vi "2013_01_05 Durability8 Main debug.vi"() -> ()   [LabVIEW 2011]
uses:
  MotorTypeDef.ctl
  <vilib>/DAQmx/write.llb/DAQmx Write (Counter Time 1Chan 1Samp).vi
  <vilib>/DAQmx/read.llb/DAQmx Read (Analog 1D Wfm NChan NSamp).vi
  <vilib>/Utility/TradDaqScaling.llb/Convert Thermistor Reading (waveform).vi
  <vilib>/DAQmx/miscellaneous.llb/DAQmx Fill In Error Info.vi
  <vilib>/measure/madcrms.llb/Averaged DC-RMS for N Chan.vi
  <vilib>/measure/NI_MAPro.lvlib
  Program Files/National Instruments/LabVIEW 2011/resource/objmgr/daqmx.rc
panel:
  out "size(s)":i32
  out "error out":errorcluster
  out "main":i32
  out "Voltages":waveform(dbl)[](graph)
  out "Currents":waveform(dbl)[](graph)
  in  "Motor 8":T1 {"Elapsed Time" format="%<%H:%M:%S>t"; "Efficiency" format="%#_3g%%"; "Supply Voltage (V)" format="%#_3f"; "Power Output (W)" format="%#_3g"; "Power Usage (W)" format="%#_3g"; "Torque (mNm)" format="%#_3g"; "RPM" scale=0.0..40000.0 scale format="%#.6p"}
  in  "Motor 7":T1 {"Elapsed Time" format="%<%H:%M:%S>t"; "Efficiency" format="%#_3g%%"; "Supply Voltage (V)" format="%#_3f"; "Power Output (W)" format="%#_3g"; "Power Usage (W)" format="%#_3g"; "Torque (mNm)" format="%#_3g"; "RPM" scale=0.0..40000.0 scale format="%#.6p"}
  in  "Motor 6":T1 {"Elapsed Time" format="%<%H:%M:%S>t"; "Efficiency" format="%#_3g%%"; "Supply Voltage (V)" format="%#_3f"; "Power Output (W)" format="%#_3g"; "Power Usage (W)" format="%#_3g"; "Torque (mNm)" format="%#_3g"; "RPM" scale=0.0..40000.0 scale format="%#.6p"}
  in  "Motor 5":T1 {"Elapsed Time" format="%<%H:%M:%S>t"; "Efficiency" format="%#_3g%%"; "Supply Voltage (V)" format="%#_3f"; "Power Output (W)" format="%#_3g"; "Power Usage (W)" format="%#_3g"; "Torque (mNm)" format="%#_3g"; "RPM" scale=0.0..40000.0 scale format="%#.6p"}
  in  "Motor 4":T1 {"Elapsed Time" format="%<%H:%M:%S>t"; "Efficiency" format="%#_3g%%"; "Supply Voltage (V)" format="%#_3f"; "Power Output (W)" format="%#_3g"; "Power Usage (W)" format="%#_3g"; "Torque (mNm)" format="%#_3g"; "RPM" scale=0.0..40000.0 scale format="%#.6p"}
  in  "Motor 3":T1 {"Elapsed Time" format="%<%H:%M:%S>t"; "Efficiency" format="%#_3g%%"; "Supply Voltage (V)" format="%#_3f"; "Power Output (W)" format="%#_3g"; "Power Usage (W)" format="%#_3g"; "Torque (mNm)" format="%#_3g"; "RPM" scale=0.0..40000.0 scale format="%#.6p"}
  in  "Motor 2":T1 {"Elapsed Time" format="%<%H:%M:%S>t"; "Efficiency" format="%#_3g%%"; "Supply Voltage (V)" format="%#_3f"; "Power Output (W)" format="%#_3g"; "Power Usage (W)" format="%#_3g"; "Torque (mNm)" format="%#_3g"; "RPM" scale=0.0..40000.0 scale format="%#.6p"}
  in  "Motor 1":T1 {"Elapsed Time" format="%<%H:%M:%S>t"; "Efficiency" format="%#_3g%%"; "Supply Voltage (V)" format="%#_3f"; "Power Output (W)" format="%#_3g"; "Power Usage (W)" format="%#_3g"; "Torque (mNm)" format="%#_3g"; "RPM" scale=0.0..40000.0 scale format="%#.6p"}
  out "Motor Temp":dbl(slide) scale=90.0..110.0
  out "Tank Temp":dbl(slide) scale=90.0..110.0
  out "RMS Voltages":waveform(dbl)[](graph)
  out "RMS Currents":waveform(dbl)[](graph)
  in  "Temp Probe\nOn Motor":dbl=1.0
  out "loop time (ms)":u32
  in  "stop":bool
  in  "Unlock PWM":bool=TRUE
  in  "PWM 2":dbl(slide)=100.0 min=0.0 max=100.0 step=5.0 scale=0.0..100.0
  in  "PWM 1":dbl(slide) min=0.0 max=100.0 step=5.0 scale=0.0..100.0
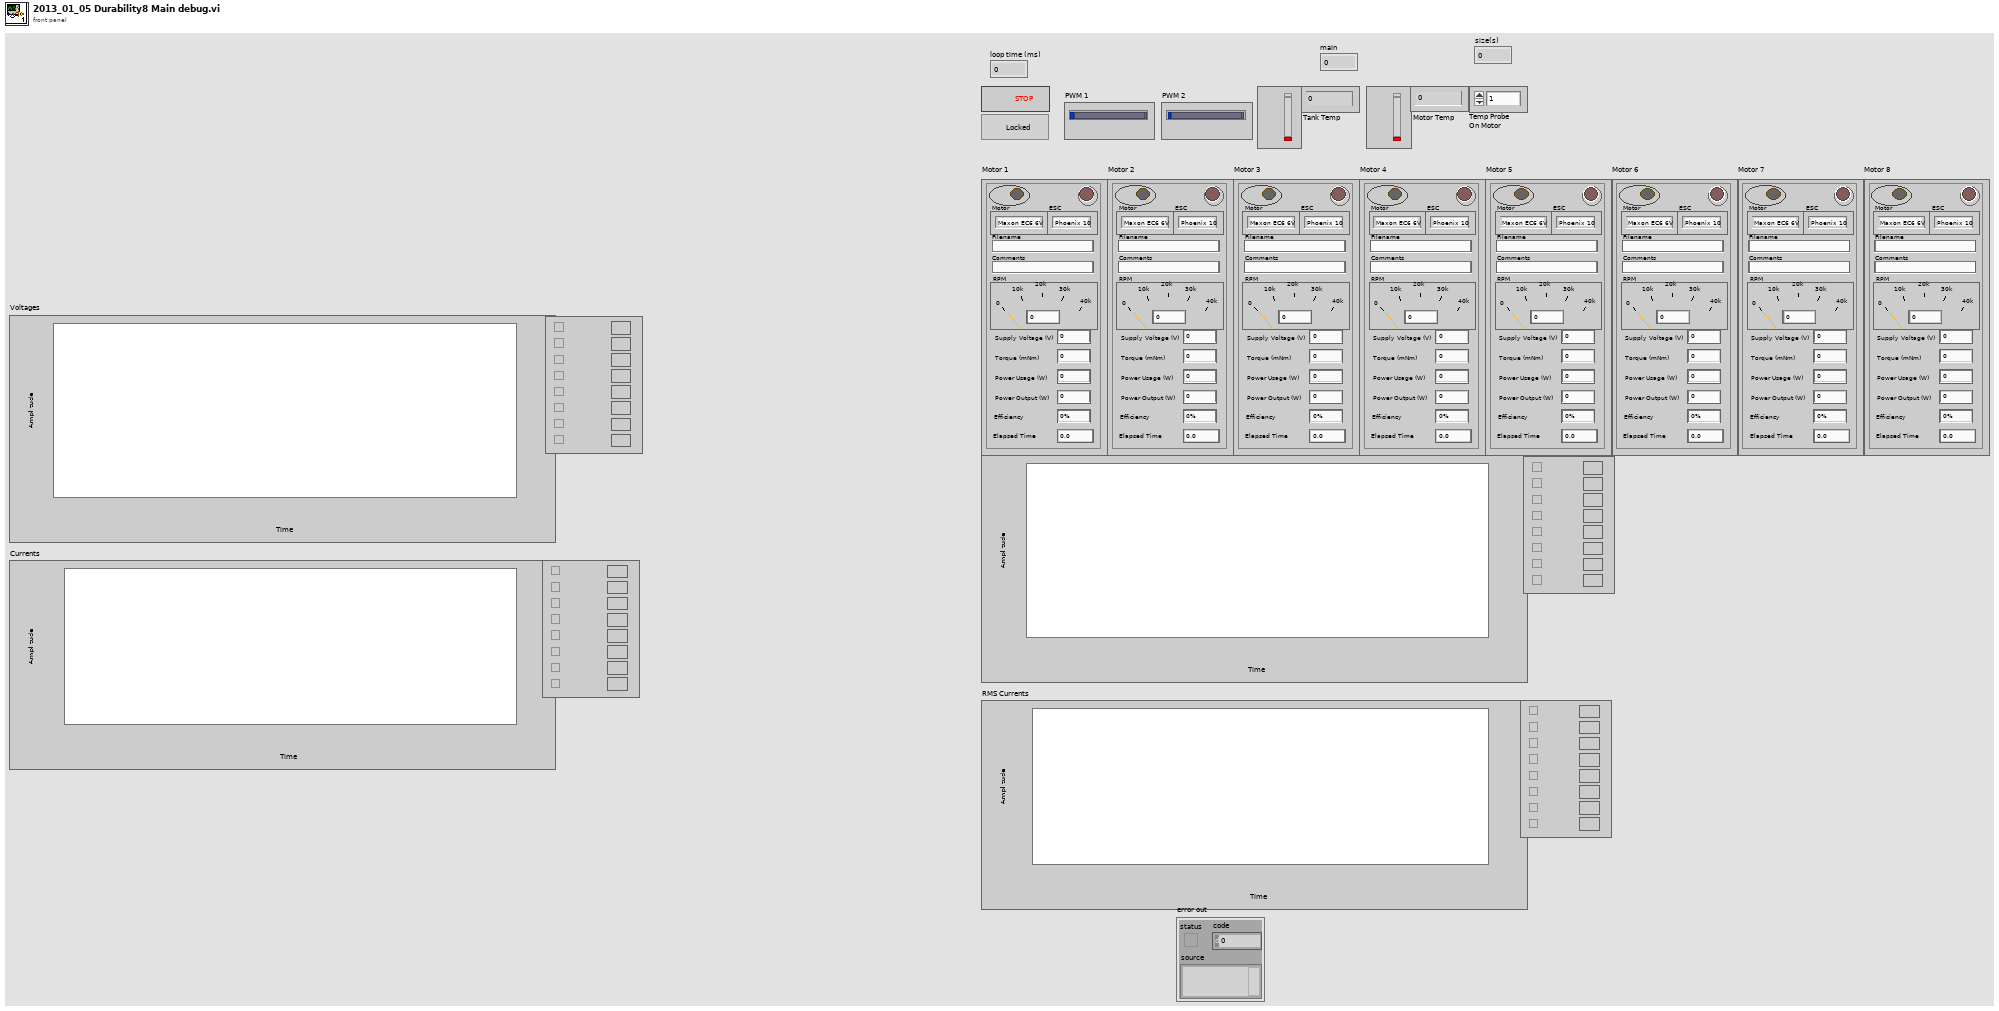
[diagram p1: front panel]
types:
  T1 = typedef "MotorTypeDef.ctl" = cluster{"Enabled":bool, "Fail":bool, "RPM":dbl, "Motor":enum16{"Maxon EC6 6V", "Maxon EC4 6V", "FH 0620 6V", "FH 0620 12V"}, "ESC":enum16{"Phoenix 10", "Maxon", "FH 1801"}, "Torque (mNm)":dbl, "Power Usage (W)":dbl, "Power Output (W)":dbl, "Supply Voltage (V)":dbl, "Efficiency":dbl, "Filename":string, "Comments":string, "Elapsed Time":dbl, "Counter":dbl}
  T2 = enum8{"Enabled", "Disabled", "Disabled and Grayed Out"}
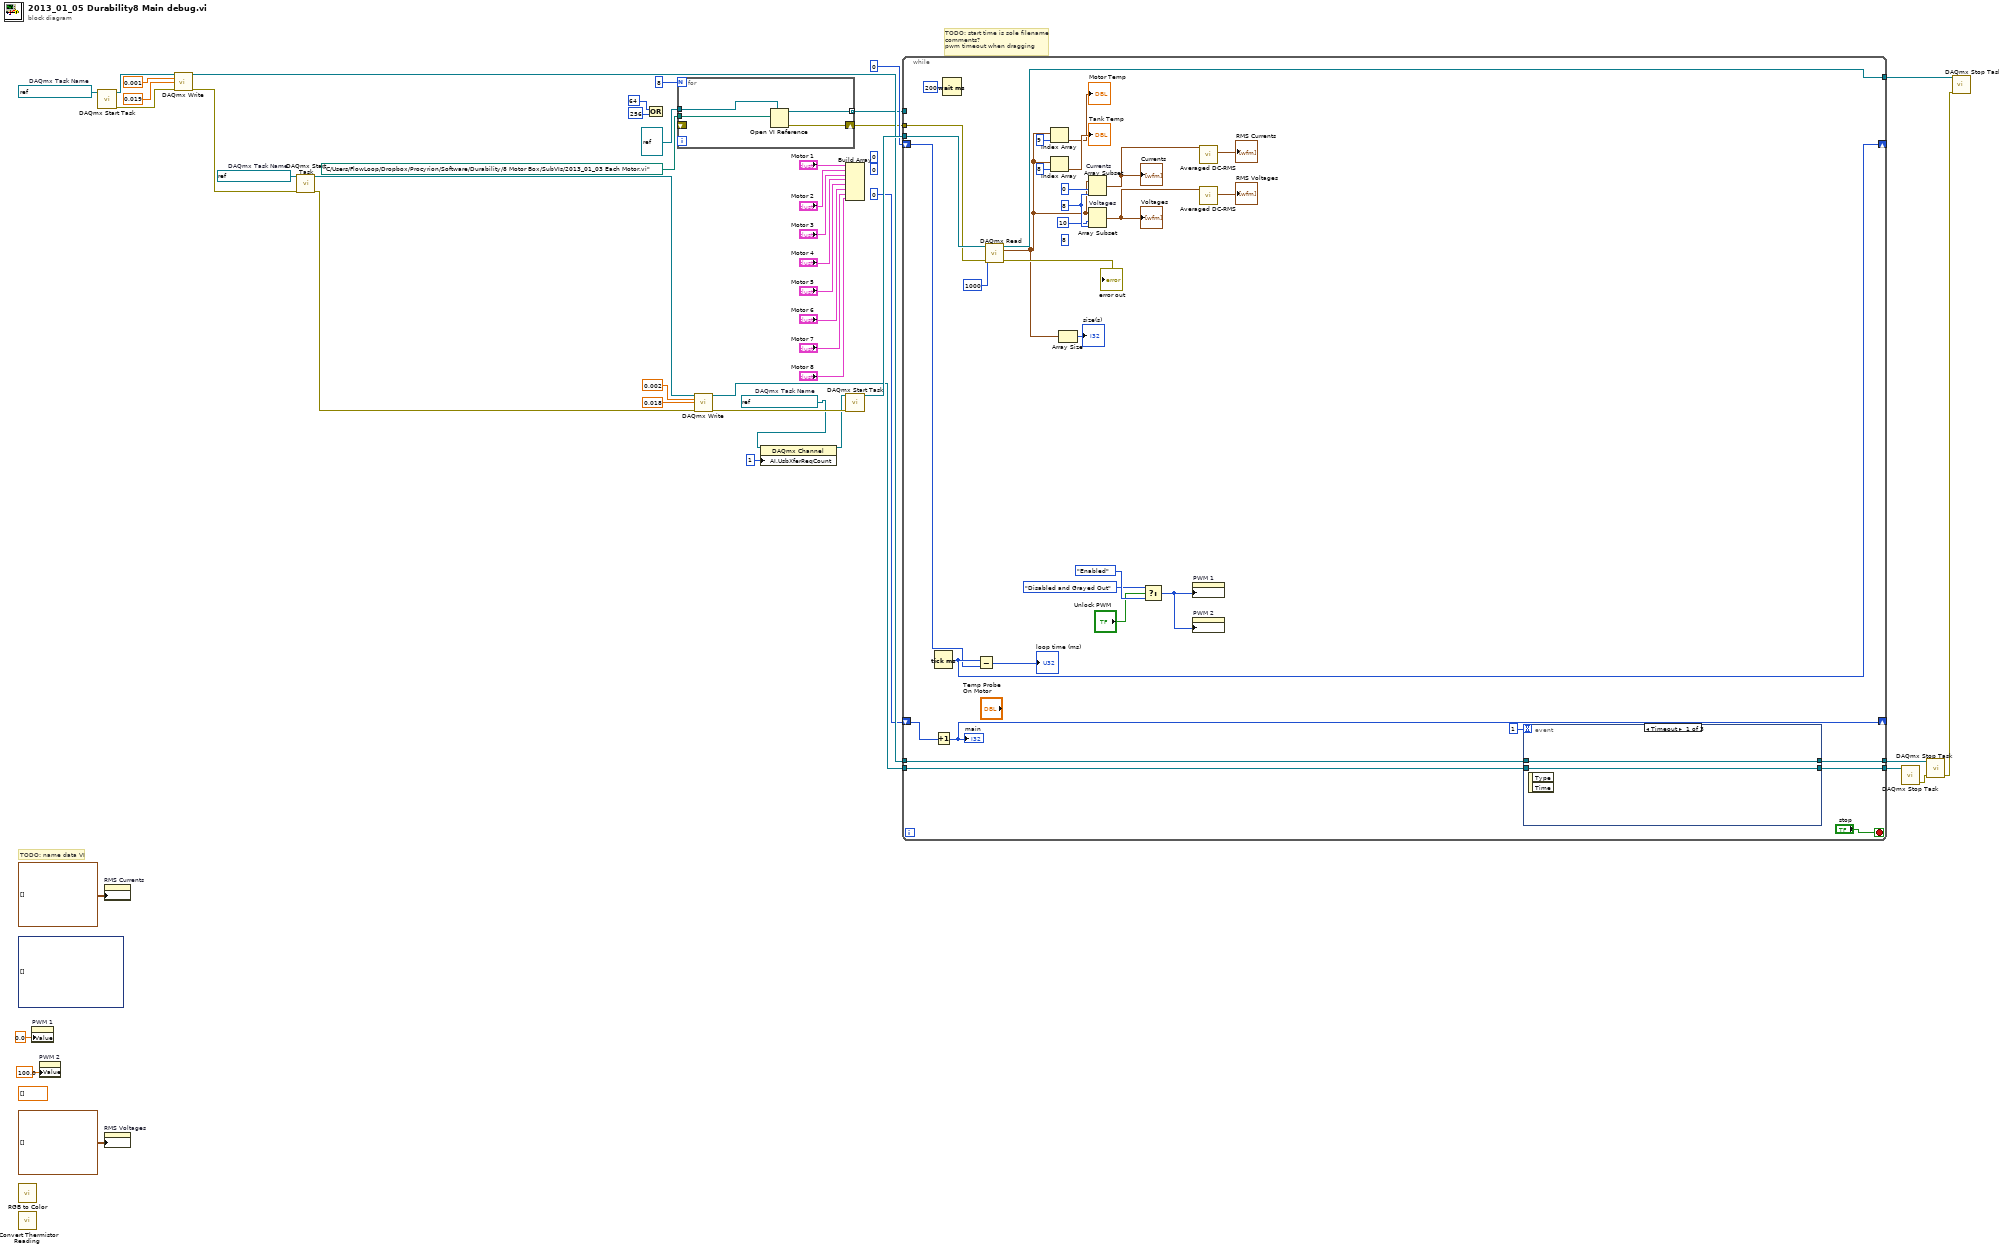
[diagram p0: block diagram]
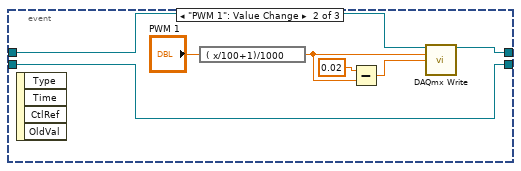
[diagram p2: hidden frame]
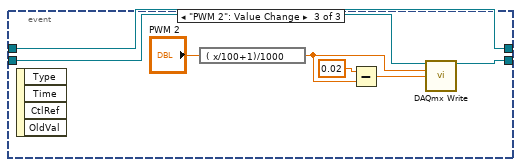
[diagram p3: hidden frame]
diagram:
  (unwired) 0 ("for")
  (unwired) 0 ("for")
  (unwired) dynamicdata[] []
  (unwired) dbl[] [] ("History Data")
  w41 = refnum<k21> "Durability8 PWM2"  # DAQmx Task Name
  w42 = refnum<k21> "Durability8 PWM1"  # DAQmx Task Name
  w2 = refnum<k21> "Durability8 Acquire"  # DAQmx Task Name
  # "TODO: start time is sole filename\ncomments?\npwm timeout when dragging"
  # "TODO: name data VI"
  n1 = call <vilib>:"RGB to Color.vi"() -> ()  [unwired: 3 in, 1 out]
  n2 = call-poly <vilib>:"Convert Thermistor Reading.vi"() -> ()  [unwired: 7 in, 1 out]
  n3 = property on="PWM 1" class="Slide (strict)"("Value"=0.0 ("PWM 1")) -> ()  [unwired: 2 in, 2 out]
  n4 = property on="PWM 2" class="Slide (strict)"("Value"=100.0 ("PWM 2")) -> ()  [unwired: 2 in, 2 out]
  n5 = call <vilib>:"DAQmx Start Task.vi"("task/channels in"=w42) -> ("task out"=w38:refnum<k21>, "error out"=w36:errorcluster)  [unwired: 13 in]
  n6 = property on="RMS Currents" class="WFChart (strict)"("History Data"=waveform(dbl)[][] []) -> ()  [unwired: 2 in, 2 out]
  n7 = property on="RMS Voltages" class="WFChart (strict)"("History Data"=waveform(dbl)[][] []) -> ()  [unwired: 2 in, 2 out]
  n8 = call-poly <vilib>:"DAQmx Write.vi"("task/channels in"=w38, "high time"=0.001 ("data"), "low time"=0.019 ("data"), "error in"=w36) -> ("task out"=w40:refnum<k21>, "error out"=w35:errorcluster)  [unwired: 9 in, 1 out]
  n9 = call <vilib>:"DAQmx Start Task.vi"("task/channels in"=w41, "error in"=w35) -> ("task out"=w37:refnum<k21>, "error out"=w34:errorcluster)  [unwired: 12 in]
  n10 = Compound Arithmetic op=OR(64 ("options"), 256 ("options")) -> ()  [unwired: 1 out]
  n11 = for {
    N: 8 -> [_]
    tunnel: path "C:/Users/FlowLoop/Dropbox/Procyrion/Software/Durability/8 Motor Box/SubVIs/2013_01_03 Each Motor.vi" -> [w48]
    tunnel: [w47] -> w16 mode=indexing
    tunnel: refnum<vi> refnum ("type specifier VI Refnum (for type only)") -> [w46]
    shift-right: [w45] -> w14
    shift-left: _ -> [_]
    n12 = Open VI Reference(type specifier VI Refnum (for type only)=w46, vi path=w48) -> (vi reference=w47:refnum<vi>, error out=w45:errorcluster)  [unwired: 4 in]
  }
  n13 = call-poly <vilib>:"DAQmx Write.vi"("task/channels in"=w37, "high time"=0.002 ("data"), "low time"=0.018 ("data"), "error in"=w34) -> ("task out"=w39:refnum<k21>, "error out"=w33:errorcluster)  [unwired: 9 in, 1 out]
  n14 = property class="DAQmx Channel"(reference=w2, "AI.UsbXferReqCount"=u32 1) -> (reference out=w1:refnum<k21>)  [unwired: 1 in, 1 out]
  n15 = Build Array("Motor 1", "Motor 2", "Motor 3", "Motor 4", "Motor 5", "Motor 6", "Motor 7", "Motor 8") -> ()  [unwired: 1 out]
  n16 = call <vilib>:"DAQmx Start Task.vi"("task/channels in"=w1, "error in"=w33) -> ("task out"=w44:refnum<k21>)  [unwired: 12 in, 1 out]
  n17 = while {
    tunnel: w44 -> [w82]
    tunnel: [w81] -> w43
    tunnel: w14 -> [w56]
    shift-right: [w76] -> _
    shift-left: u32 0 ("millisecond timer value") -> [w75]
    tunnel: w40 -> [w63]
    tunnel: w39 -> [w62]
    tunnel: [w61] -> w32
    tunnel: [w60] -> w23
    tunnel: w16 -> [_]
    shift-right: [w54] -> _
    shift-left: 0 ("for") -> [w55]
    stop <- "stop" stop-if-true
    (unwired) 8
    w71 = 8 ("length")
    n18 = Tick Count (ms)() -> (millisecond timer value=w76:u32)
    n19 = Increment(x=w55) -> (x+1=w54:i32)
    "main" <- w54
    n20 = Wait (ms)(milliseconds to wait=u32 200) -> ()  [unwired: 1 out]
    n21 = Subtract(x=w76, y=w75) -> (x-y=→"loop time (ms)":u32)
    n22 = call-poly <vilib>:"DAQmx Read.vi"("task/channels in"=w82, "number of samples per channel"=1000, "error in"=w56) -> ("task out"=w81:refnum<k21>, "data"=w52:waveform(dbl)[], "error out"=→"error out":errorcluster)  [unwired: 10 in]
    n23 = Index Array(array=w52, index=9) -> (element=→"Motor Temp":waveform(dbl))
    n24 = Index Array(array=w52, index=8) -> (element=→"Tank Temp":waveform(dbl))
    n25 = Array Size(array=w52) -> (size(s)=→"size(s)":i32)
    n26 = Array Subset "Currents"(array=w52, index=0, length=w71) -> (w58:waveform(dbl)[])
    "Currents" <- w58
    n27 = Array Subset "Voltages"(array=w52, index=10 ("length"), length=w71) -> (w57:waveform(dbl)[])
    "Voltages" <- w57
    n28 = Select(t=T2."Disabled and Grayed Out" ("Disabled"), s="Unlock PWM", f=T2."Enabled" ("Disabled")) -> (s? t:f=w80:T2)
    n29 = property on="PWM 1" class="Slide (strict)"("DisabledEnum"=w80) -> ()  [unwired: 2 in, 2 out]
    n30 = property on="PWM 2" class="Slide (strict)"("DisabledEnum"=w80) -> ()  [unwired: 2 in, 2 out]
    n31 = call-poly <vilib>:"Averaged DC-RMS.vi"("signals in"=w58) -> ("RMS value waveforms"=→"RMS Currents":waveform(dbl)[])  [unwired: 6 in, 4 out]
    n32 = call-poly <vilib>:"Averaged DC-RMS.vi"("signals in"=w57) -> ("RMS value waveforms"=→"RMS Voltages":waveform(dbl)[])  [unwired: 6 in, 4 out]
    n33 = event shown="[0] Timeout" {
      selector: _ -> [_ _ _]
      dyn-events: _ -> [_ _ _]
      timeout: 1 -> [_ _ _]
      tunnel: w63 -> [w84 w87 w93]
      tunnel: w62 -> [w83 w85 w92]
      tunnel: [w84 w86 w93] -> w61
      tunnel: [w83 w85 w94] -> w60
      event Timeout {
        n34 = event-data() -> ()  [unwired: 1 in, 2 out]
      }
      event "PWM 1": Value Change {
        n35 = event-data() -> ()  [unwired: 1 in, 4 out]
        n36 = expression code="( x/100+1)/1000"("PWM 1") -> (w88:dbl)
        n37 = Subtract(x=0.02 ("y"), y=w88) -> (x-y=w89:dbl)
        n38 = call-poly <vilib>:"DAQmx Write.vi"("task/channels in"=w87, "high time"=w88, "low time"=w89) -> ("task out"=w86:refnum<k21>)  [unwired: 10 in, 2 out]
      }
      event "PWM 2": Value Change {
        n39 = event-data() -> ()  [unwired: 1 in, 4 out]
        n40 = expression code="( x/100+1)/1000"("PWM 2") -> (w98:dbl)
        n41 = Subtract(x=0.02, y=w98) -> (x-y=w96:dbl)
        n42 = call-poly <vilib>:"DAQmx Write.vi"("task/channels in"=w92, "high time"=w98, "low time"=w96) -> ("task out"=w94:refnum<k21>)  [unwired: 10 in, 2 out]
      }
    }
  }
  n43 = call <vilib>:"DAQmx Stop Task.vi"("task/channels in"=w23) -> ("error out"=w31:errorcluster)  [unwired: 13 in, 1 out]
  n44 = call <vilib>:"DAQmx Stop Task.vi"("task/channels in"=w32, "error in"=w31) -> ("error out"=w30:errorcluster)  [unwired: 12 in, 1 out]
  n45 = call <vilib>:"DAQmx Stop Task.vi"("task/channels in"=w43, "error in"=w30) -> ()  [unwired: 12 in, 2 out]
